vi "Actor Core.vi"(8 "error in":errorcluster, 11 "Syringe in":refnum<class "Syringe.lvclass">) -> (0 "error out":errorcluster, 3 "Actor out":refnum<class "Actor.lvclass">)   [LabVIEW 2015, in "AMS UI.lvlib" / "Syringe.lvclass"]
doc: "(<B>Filename</B>: Actor Framework.lvlib:Actor.lvclass:Actor Core.vi)\n\nReceives messages to the actor, reacts to them, and initiates any error handling that may shut the actor down.\n\nDescendant classes may override this VI to append parallel tasks for the actor to complete while it handles messages. Overrides use the Call Parent Method node."
uses:
  Syringe.lvclass
  <vilib>/ActorFramework/Actor/Actor.lvclass
  <vilib>/ActorFramework/Message Enqueuer/Message Enqueuer.lvclass/Message Enqueuer.ctl
  <vilib>/ActorFramework/Message Enqueuer/Enqueue.vi
  <vilib>/ActorFramework/Message Priority Queue/Priority Enqueue.vi
  AMS Gas Actor/AMS Gas Actor.lvclass
  Syringe Messages/Indicate Syringe Line/Indicate Syringe Line Msg.lvclass
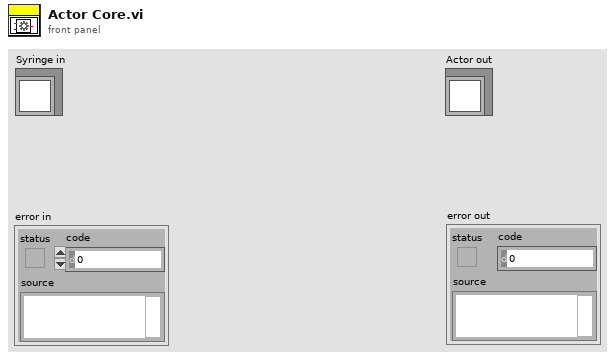
[diagram p1: front panel]
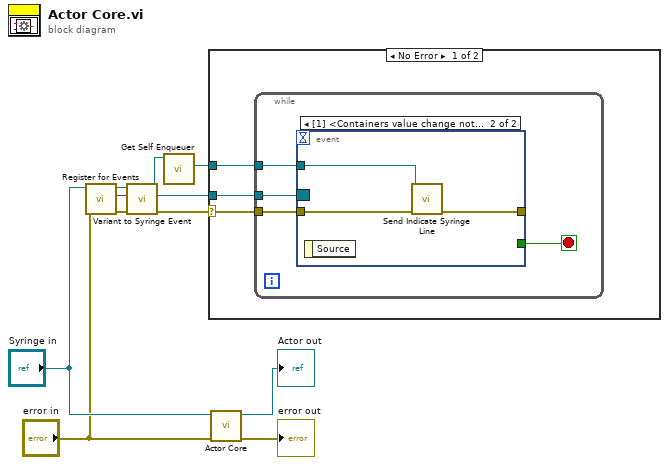
[diagram p0: block diagram]
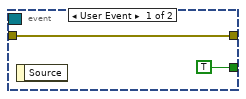
[diagram p2: hidden frame]
diagram:
  n1 = call-dynamic "Register for Events.vi"("error in (no error)"="error in", "Syringe in"="Syringe in") -> ("error out"=w7:errorcluster, "Event Registration Refnum"=w5:variant, "Syringe out"=w6:refnum<class "Syringe.lvclass">)  [unwired: 7 in]
  n2 = call "Variant to Syringe Event.vi"("error in (no error)"=w7, "variant"=w5, "Syringe in"=w6) -> ("error out"=w4:errorcluster, "Event Registration Refnum"=w3:refnum<event-registration>, "Syringe out"=w2:refnum<class "Syringe.lvclass">)  [unwired: 6 in]
  n3 = call-dynamic "Get Self Enqueuer.vi"("eActor in"=w2) -> ("Actor Framework:Message Enqueuer"=w1:refnum<class "Message Enqueuer.lvclass">)  [unwired: 9 in, 1 out]
  n4 = case shown="No Error" w4 {
    selector: w4 -> [w13 _]
    tunnel: w3 -> [w14 _]
    tunnel: w1 -> [w12 _]
    frame No Error {
      n5 = while {
        tunnel: w14 -> [w18]
        tunnel: w13 -> [w17]
        tunnel: w12 -> [w15]
        stop <- w16 stop-if-true
        n6 = event shown="[1] <Containers value change notification>: User Event" {
          selector: w18 -> [_ _]
          dyn-events: _ -> [_ _]
          timeout: _ -> [_ _]
          tunnel: w17 -> [w19 w23]
          tunnel: [w19 w22] -> _
          tunnel: [TRUE _] -> w16
          tunnel: w15 -> [_ w21]
          event User Event {
            n7 = event-data() -> ()  [unwired: 1 in, 1 out]
          }
          event User Event {
            n8 = event-data() -> ()  [unwired: 1 in, 1 out]
            n9 = call "Send Indicate Syringe Line.vi"("error in (no error)"=w23, "Message Enqueuer"=w21) -> ("error out"=w22:errorcluster)  [unwired: 8 in, 1 out]
          }
        }
      }
    }
    frame Error {
    }
  }
  n10 = call-parent "Actor Core.vi"("error in"="error in", "Actor in"="Syringe in") -> ("error out"=→"error out":errorcluster, "Actor out"=→"Actor out":refnum<class "Actor.lvclass">)  [unwired: 8 in]
